vi "MOCKBEAR_Initialize.vi"(8 "error in (no error)":errorcluster, 11 "MOCKBEAR in":refnum<class "MOCKBEAR.lvclass">) -> (0 "error out":errorcluster, 3 "MOCKBEAR out":refnum<class "MOCKBEAR.lvclass">)   [LabVIEW 2021, in "MOCKBEAR.lvclass"]
uses:
  MOCKBEAR.lvclass
  MOCKBEAR.lvclass/MOCKBEAR.ctl
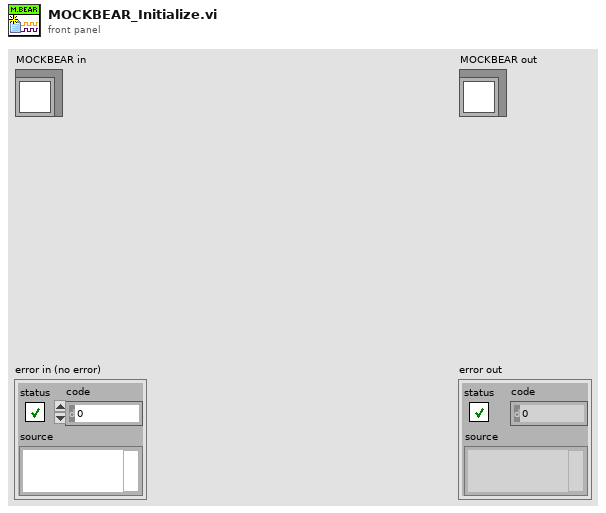
[diagram p1: front panel]
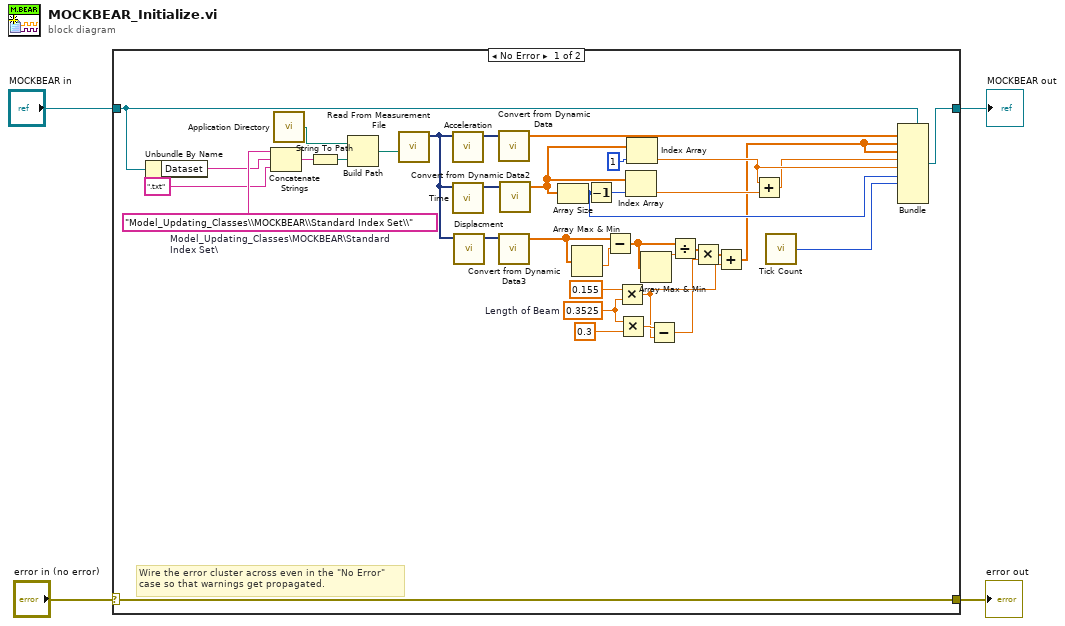
[diagram p0: block diagram]
diagram:
  n1 = case shown="No Error" "error in (no error)" {
    selector: "error in (no error)" -> [w40 w42]
    tunnel: [w40 w42] -> w3
    tunnel: [w15 w41] -> w1
    tunnel: "MOCKBEAR in" -> [w17 w41]
    frame No Error {
      w21 = "Model_Updating_Classes\\MOCKBEAR\\Standard Index Set\\"  # Model_Updating_Classes\MOCKBEAR\Standard Index Set\
      w29 = 0.3525  # Length of Beam
      # "Wire the error cluster across even in the \"No Error\"\ncase so that warnings get propagated."
      n2 = Unbundle By Name(w17) -> ("Dataset"=w20:string)
      n3 = Concatenate Strings(w21, w20, ".txt") -> (w6:string)
      n4 = call <vilib>:"Application Directory.vi"() -> ("Application Directory"=w14:path)
      n5 = String To Path(string=w6) -> (path=w18:path)
      n6 = Build Path(base path=w14, name or relative path=w18) -> (appended path=w39:path)
      n7 = call "Read From Measurement File"("Filename"=w39) -> ("Signals"=w32:dynamicdata)  [unwired: 5 in, 5 out]
      n8 = call "Acceleration"("Signals"=w32) -> ("Signal Out"=w37:dynamicdata)  [unwired: 9 in, 1 out]
      n9 = call "Time"("Signals"=w32) -> ("Signal Out"=w36:dynamicdata)  [unwired: 9 in, 1 out]
      n10 = call "Displacment"("Signals"=w32) -> ("Signal Out"=w31:dynamicdata)  [unwired: 9 in, 1 out]
      n11 = call "Convert from Dynamic Data"("Dynamic Data Type"=w37) -> ("Array"=w16:dbl[])  [unwired: 3 in]
      n12 = call "Convert from Dynamic Data3"("Dynamic Data Type"=w31) -> ("Array"=w25:dbl[])  [unwired: 3 in]
      n13 = call "Convert from Dynamic Data2"("Dynamic Data Type"=w36) -> ("Array"=w34:dbl[])  [unwired: 3 in]
      n14 = Array Size(array=w34) -> (size(s)=w9:i32)
      n15 = Array Max & Min(array=w25) -> (min value=w27:dbl)  [unwired: 3 out]
      n16 = Decrement(x=w9) -> (x-1=w33:i32)
      n17 = Subtract(x=w25, y=w27) -> (x-y=w24:dbl[])
      n18 = Multiply(x=0.155, y=w29) -> (x*y=w12:dbl)
      n19 = Multiply(x=w29, y=0.3) -> (x*y=w13:dbl)
      n20 = Index Array(array=w34, index=w33) -> (element=w38:dbl)
      n21 = Index Array(array=w34, index=1) -> (element=w8:dbl)
      n22 = Array Max & Min(array=w24) -> (max value=w23:dbl)  [unwired: 3 out]
      n23 = Subtract(x=w13, y=w12) -> (x-y=w11:dbl)
      n24 = Divide(x=w24, y=w23) -> (x/y=w22:dbl[])
      n25 = Multiply(x=w22, y=w11) -> (x*y=w26:dbl[])
      n26 = Add(x=w26, y=w12) -> (x+y=w5:dbl[])
      n27 = Add(x=w8, y=w38) -> (x+y=w7:dbl)
      n28 = call "Tick Count"() -> ("Tick Count(uSec)"=w10:u32)
      n29 = Bundle(cluster=w17, w16, w5, w5, w7, w8, w9, w10) -> (w15:refnum<class "MOCKBEAR.lvclass">)  [unwired: 3 in]
    }
    frame Error {
    }
  }
  "error out" <- w3
  "MOCKBEAR out" <- w1
